vi "Test Edge Component Drag.vi"(0 "FSM.Graph In":refnum<class "FSM.Graph.lvclass">, 7 "Coords":T1) -> (4 "FSM.Graph Out":refnum<class "FSM.Graph.lvclass">, 8 "label drag?":bool, 14 "attached node":string, 15 "drag control?":bool)   [LabVIEW 2020, in "FSM.Graph.lvclass"]
uses:
  FSM.Graph.lvclass
  <vilib>/Utility/miscctls.llb/LVPoint32TypeDef.ctl
  FSM.Graph.lvclass/FSM.Graph.ctl
  FSM.Edge/FSM.Edge.lvclass
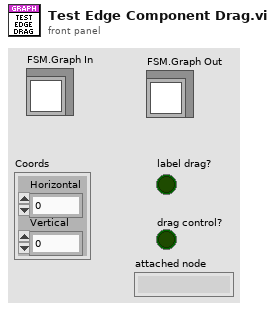
[diagram p1: front panel]
types:
  T1 = typedef "LVPoint32TypeDef.ctl" = cluster{"Horizontal":i32, "Vertical":i32}
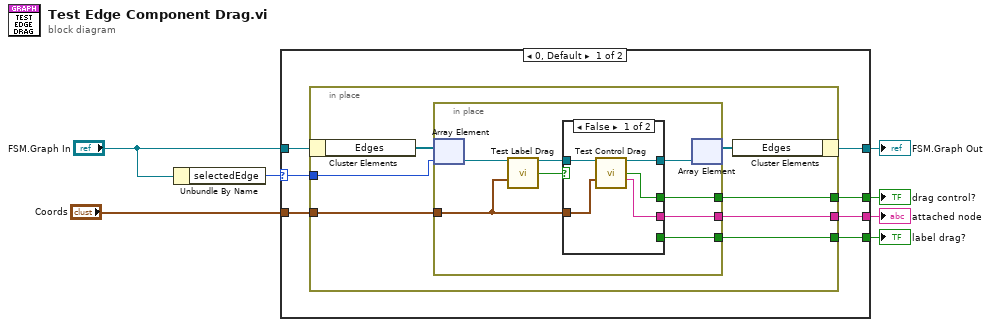
[diagram p0: block diagram]
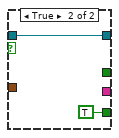
[diagram p2: hidden frame]
diagram:
  n1 = Unbundle By Name("FSM.Graph In") -> ("selectedEdge"=w6:i32)
  n2 = case shown="0, Default" w6 {
    selector: w6 -> [w12 _]
    tunnel: "Coords" -> [w14 _]
    tunnel: "FSM.Graph In" -> [w13 w37]
    tunnel: [w11 w37] -> w4
    tunnel: [w10 _] -> w3
    tunnel: [w9 _] -> w2
    tunnel: [w8 _] -> w1
    frame 0, Default {
      n3 = in-place {
        in-place-border: w14 -> [w21]
        in-place-border: w12 -> [w19]
        in-place-border: [w17] -> w10
        in-place-border: [w16] -> w9
        in-place-border: [w15] -> w8
        n4 = in-place-cluster #1(w13) -> ("Edges"=w20:refnum<class "FSM.Edge.lvclass">[])
        n5 = in-place {
          in-place-border: w21 -> [w26]
          in-place-border: [w24] -> w17
          in-place-border: [w23] -> w16
          in-place-border: [w22] -> w15
          n6 = in-place-array #2(w20, w19) -> (w29:refnum<class "FSM.Edge.lvclass">)
          n7 = call "Test Label Drag.vi"("FSM.Edge In"=w29, "Coords"=w26) -> ("FSM.Edge Out"=w27:refnum<class "FSM.Edge.lvclass">, "drag label?"=w28:bool)  [unwired: 12 in]
          n8 = case shown="False" w28 {
            tunnel: w27 -> [w34 w36]
            tunnel: w26 -> [w33 _]
            tunnel: [w32 w36] -> w25
            tunnel: [_ TRUE] -> w24
            tunnel: [w31 _] -> w23
            tunnel: [w30 _] -> w22
            frame False {
              n9 = call "Test Control Drag.vi"("FSM.Edge In"=w34, "Coords"=w33) -> ("FSM.Edge Out"=w32:refnum<class "FSM.Edge.lvclass">, "drag control?"=w31:bool, "attached node"=w30:string)  [unwired: 11 in]
            }
            frame True {
            }
          }
          n10 = in-place-array #2(w25) -> (w18:refnum<class "FSM.Edge.lvclass">[])  [unwired: 1 out]
        }
        n11 = in-place-cluster #1("Edges"=w18) -> (w11:refnum<class "FSM.Graph.lvclass">)
      }
    }
    frame -1 {
    }
  }
  "FSM.Graph Out" <- w4
  "label drag?" <- w3
  "drag control?" <- w2
  "attached node" <- w1
